vi "Spawn.vi"(4 "Persistent Layers":refnum<class "Actor.lvclass">[](array[class]), 6 "Root":bool, 9 "UID":string, 10 "Unified Actor":refnum<class "Actor.lvclass">, 11 "TEMPLATE Actor in":refnum<class "TEMPLATE Actor.lvclass">) -> (0 "Error out":errorcluster, 3 "TEMPLATE Actor out":refnum<class "TEMPLATE Actor.lvclass">)   [LabVIEW 2025, in "_Template.lvlib" / "Templates.lvlib" / "TEMPLATE Actor.lvlib" / "TEMPLATE Actor.lvclass"]
uses:
  TEMPLATE Actor.lvclass
  jettl/jettl/Actor/Actor.lvclass
  TEMPLATE Actor.lvclass/TEMPLATE Actor.ctl
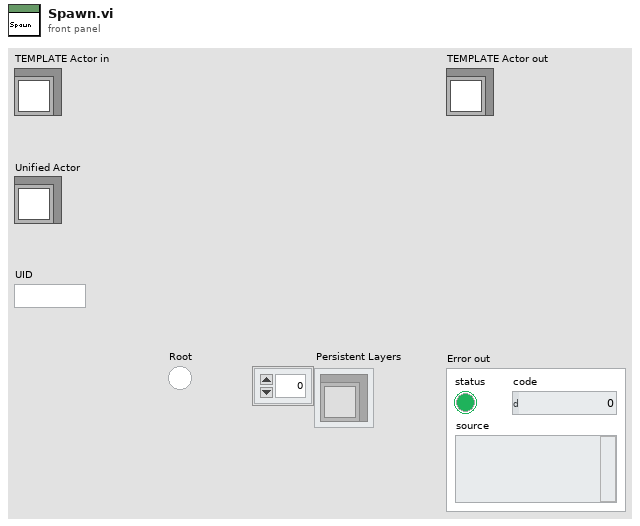
[diagram p1: front panel]
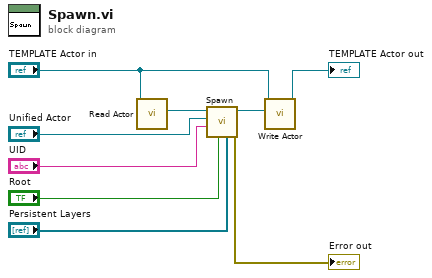
[diagram p0: block diagram]
diagram:
  n1 = call-dynamic "Read Actor.vi"("TEMPLATE Actor in"="TEMPLATE Actor in") -> ("Actor"=w6:refnum<class "Actor.lvclass">)  [unwired: 10 in]
  n2 = call-dynamic "Spawn.vi"("Persistent Layers"="Persistent Layers", "Root"="Root", "UID"="UID", "Unified Actor"="Unified Actor", "Actor in"=w6) -> ("Error out"=→"Error out":errorcluster, "Actor out"=w4:refnum<class "Actor.lvclass">)  [unwired: 5 in]
  n3 = call-dynamic "Write Actor.vi"("Actor"=w4, "TEMPLATE Actor in"="TEMPLATE Actor in") -> ("TEMPLATE Actor out"=→"TEMPLATE Actor out":refnum<class "TEMPLATE Actor.lvclass">)  [unwired: 9 in]
